vi "Read Bookmarks.vi"(8 "error in (no error)":errorcluster, 11 "Word_Report in":refnum<class "Word_Report.lvclass">) -> (0 "error out":errorcluster, 2 "Bookmarks":string[](array[string]), 3 "Word_Report out":refnum<class "Word_Report.lvclass">)   [LabVIEW 2018, in "WordReportGeneration.lvlib" / "Word_Report.lvclass"]
uses:
  Word_Report.lvclass
  Word_Report.lvclass/Word_Report.ctl
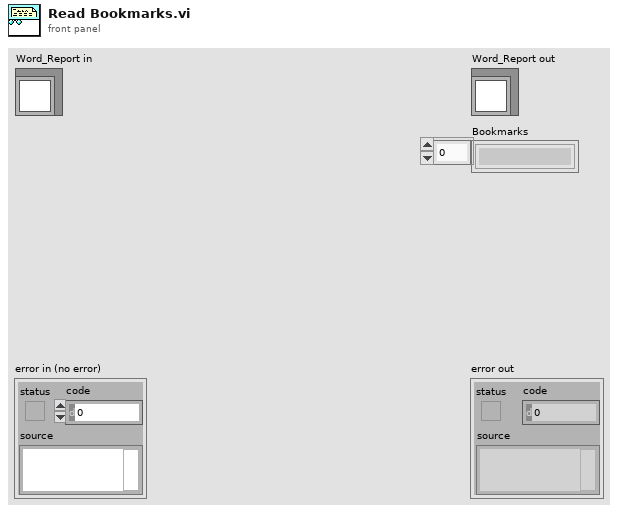
[diagram p1: front panel]
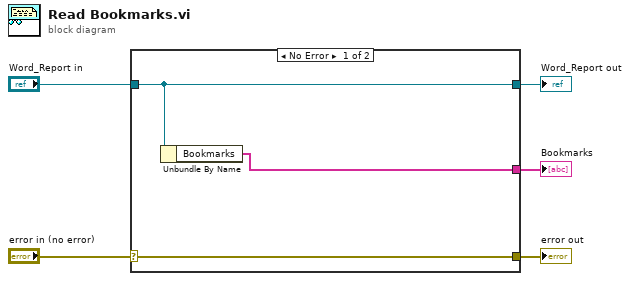
[diagram p0: block diagram]
diagram:
  n1 = case shown="No Error" "error in (no error)" {
    selector: "error in (no error)" -> [w8 w9]
    tunnel: [w8 w9] -> w4
    tunnel: [w7 w10] -> w2
    tunnel: "Word_Report in" -> [w7 w10]
    tunnel: [w6 _] -> w1
    frame No Error {
      n2 = Unbundle By Name(w7) -> ("Bookmarks"=w6:string[])
    }
    frame Error {
    }
  }
  "error out" <- w4
  "Word_Report out" <- w2
  "Bookmarks" <- w1
